vi "Get_Trigger_Output_Mode.vi"(8 "error in (no error)":errorcluster, 11 ".NET Reference in":refnum<k24>) -> (0 "error out":errorcluster, 2 "mode":enum16{"None", "Stop", "Start", "Step", ""}(ring), 3 ".NET Reference out":refnum<k24>)   [LabVIEW 2017]
uses:
  LV_IL_Sample/DLL/InstrumentDLL.dll
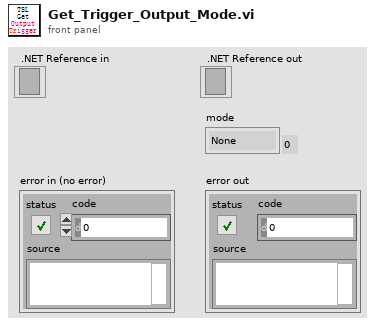
[diagram p1: front panel]
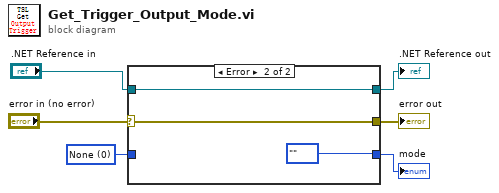
[diagram p0: block diagram]
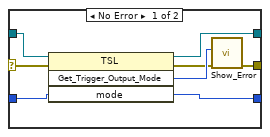
[diagram p2: hidden frame]
diagram:
  w2 = 0 items=["None", "Stop", "Start", "Step"] ("mode")
  n1 = case shown="Error" "error in (no error)" {
    selector: "error in (no error)" -> [w10 w16]
    tunnel: [w7 w16] -> w6
    tunnel: [w14 w17] -> w5
    tunnel: [w13 enum16{"None", "Stop", "Start", "Step", ""}."" ("mode")] -> w4
    tunnel: ".NET Reference in" -> [w12 w17]
    tunnel: w2 -> [w11 _]
    frame No Error {
      n2 = invoke on="调用节点" class="TSL" method="Get_Trigger_Output_Mode"(reference=w12, error in=w10, "mode"=w11) -> (reference out=w14:refnum<k24>, error out=w8:errorcluster, "Get_Trigger_Output_Mode"=w9:i32, "mode"=w13:i32)  [unwired: 1 in]
      n3 = call "Show_Error.vi"("error in (no error)"=w8, "Error"=w9) -> ("error out"=w7:errorcluster)  [unwired: 9 in]
    }
    frame Error {
    }
  }
  "error out" <- w6
  ".NET Reference out" <- w5
  "mode" <- w4
